vi "Lab3_ASK.vi"() -> ()   [LabVIEW 2019]
uses:
  <vilib>/addons/Modulation/Digital/General/MT Generate Bits (Galois, PN Order).vi
  <vilib>/addons/Modulation/Digital/Support/Common/Validators/mod_Generate Bits Validate.vi
  <vilib>/addons/Modulation/Analog/support/mod_Set Error Source.vi
  <vilib>/addons/Modulation/Digital/Support/Common/Validators/mod_AWGN Validate.vi
  <vilib>/addons/Modulation/Digital/Impairments/subVIs/mod_createSeeds.vi
  <vilib>/addons/Modulation/Digital/Support/Common/Validators/mod_Validate Samples Per Symbol.vi
  <vilib>/addons/Modulation/Analog/support/Validators/mod_Validate Complex Waveform.vi
  <vilib>/addons/Modulation/Analog/support/Validators/mod_WFErrorHandler.vi
  <vilib>/addons/Modulation/Digital/General/MT Generate ASK system parameters (M).vi
  <vilib>/addons/Modulation/Digital/General/subVIs/mod_Generate Bits PN Sequence.vi
  <vilib>/addons/Modulation/Digital/Support/Common/Validators/mod_Generate Filter Coefficients Validate.vi
  <vilib>/addons/Modulation/Digital/General/subVIs/mod_Generate Filter Coefficients.vi
  <vilib>/Analysis/1siggen.llb/Gaussian White Noise (obs 90).vi
  <vilib>/addons/Modulation/Analog/MT Upconvert Baseband (Real).vi
  <vilib>/addons/Modulation/niDMT.lvlib
  <vilib>/addons/Modulation/niAMT.lvlib
panel:
  out "Upconverted Wave":waveform(dbl)(graph)
  in  "Reset":bool=TRUE
  out "Waveform Graph":cluster{"t0":dbl, "dt":dbl, "Y":dbl[]}(graph)
  in  "Symbol Rate(HZ)":dbl format="%#_2p"
  in  "Carrier Freq(HZ)":dbl format="%#_2p"
  in  "pulse shaping filter":T1(ring)
  in  "M-ASK":u16(ring) items=["2"=2, "4"=4, "8"=8, "16"=16]
  in  "Eb/No(dB)":dbl
  in  "stop":bool
  out "ASK Constellation":T2(graph)
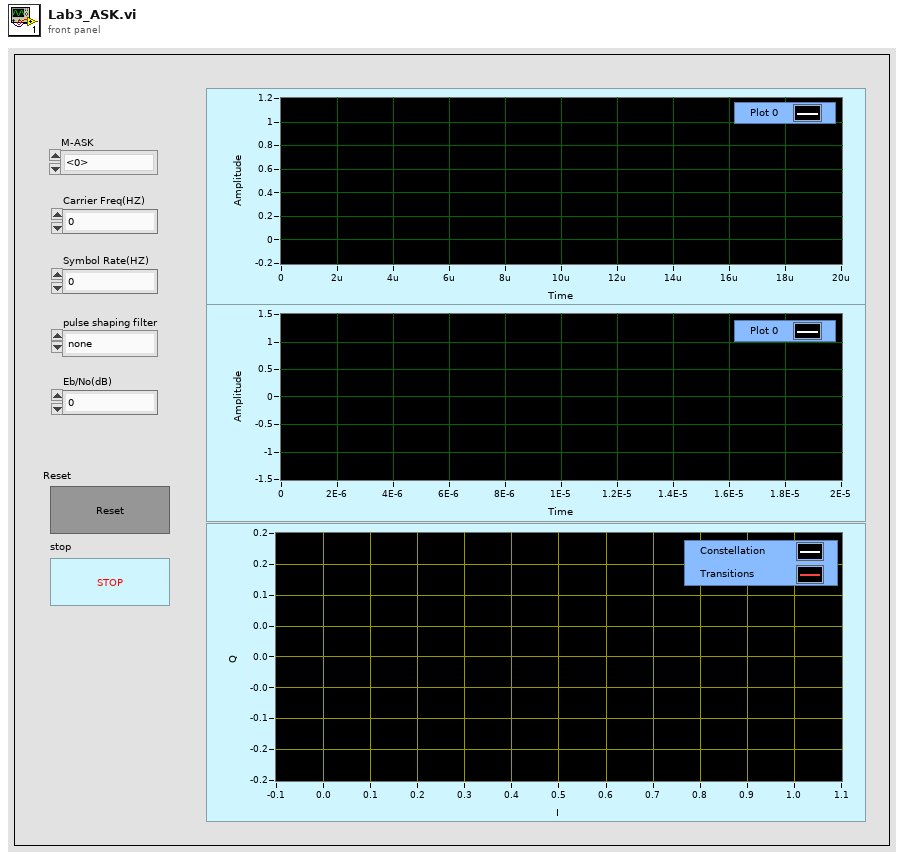
[diagram p1: front panel]
types:
  T1 = enum16{"none", "Raised Cosine", "Root Raised Cos", "Gaussian"}
  T2 = cluster{"Decimated Array":dbl[], "Decimated Array":dbl[]}[]
  T3 = enum16{"FSK", "PSK", "QAM", "MSK", "PAM", "ASK", "CPM"}
  T4 = cluster{"samples per symbol (16)":i32, "symbol map":cdb[]}
  T5 = typedef "niAMT.lvlib/Complex Data Waveform.ctl" = cluster{"t0":dbl, "dt":dbl, "Y":cdb[]}
  T6 = cluster{"constellation":dbl[], "oversampled data":dbl[]}[]
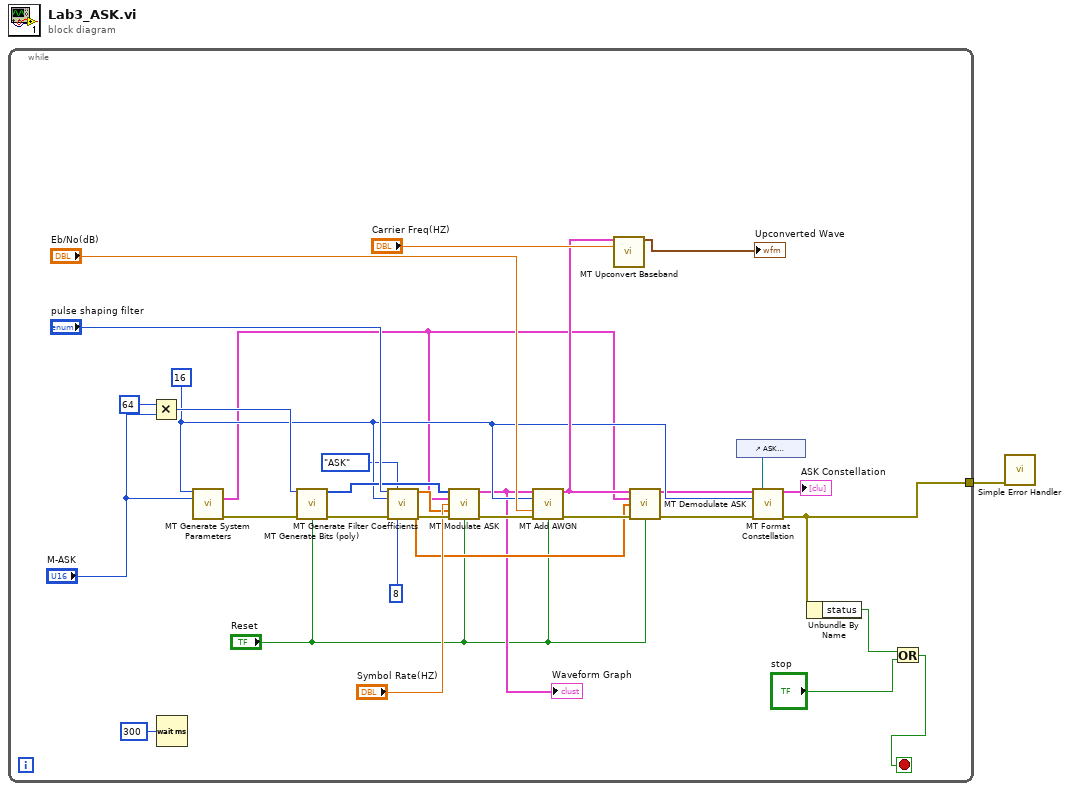
[diagram p0: block diagram]
diagram:
  n1 = while {
    tunnel: [w9] -> w1
    stop <- w6 stop-if-true
    w13 = 16 ("samples per symbol (16)")
    n2 = Multiply(x=u16 64, y="M-ASK") -> (x*y=w25:u16)
    n3 = Wait (ms)(milliseconds to wait=u32 300) -> ()  [unwired: 1 out]
    n4 = call-poly <vilib>:"MT Generate System Parameters.vi"("samples per symbol (16)"=w13, "M-ASK (2)"="M-ASK") -> ("ASK system parameters"=w12:T4, "error out"=w29:errorcluster)  [unwired: 11 in, 1 out]
    n5 = call-poly <vilib>:"MT Generate Bits (poly).vi"("total bits (128)"=w25, "error in (no error)"=w29, "reset? (T)"="Reset") -> ("output bit stream"=w14:i8[], "error out"=w28:errorcluster)  [unwired: 10 in, 1 out]
    n6 = call <vilib>:"MT Generate Filter Coefficients.vi"("pulse shaping filter (none)"="pulse shaping filter", "modulation type"=T3."ASK", "pulse shaping samples per symbol (16)"=w13, "error in (no error)"=w28, "filter length (symbols)"=8) -> ("pulse shaping filter coefficients"=w16:dbl[], "matched filter coefficients"=w17:dbl[], "error out"=w22:errorcluster)  [unwired: 8 in]
    n7 = call <vilib>:"MT Modulate ASK.vi"("input bit stream"=w14, "ASK system parameters"=w12, "symbol rate (Hz)"="Symbol Rate(HZ)", "pulse shaping filter coefficients"=w16, "error in (no error)"=w22, "reset? (T)"="Reset") -> ("output complex waveform"=w10:T5, "error out"=w21:errorcluster)  [unwired: 7 in, 1 out]
    "Waveform Graph" <- w10
    n8 = call <vilib>:"MT Add AWGN.vi"("input complex waveform"=w10, "samples per symbol (16)"=w13, "Eb/N0 (10 dB)"="Eb/No(dB)", "error in (no error)"=w21, "reset? (T)"="Reset") -> ("output complex waveform"=w19:T5, "error out"=w18:errorcluster)  [unwired: 8 in, 1 out]
    n9 = call-poly <vilib>:"MT Upconvert Baseband.vi"("baseband waveform (complex)"=w19, "carrier frequency (Hz)"="Carrier Freq(HZ)") -> ("passband waveform"=→"Upconverted Wave":waveform(dbl))  [unwired: 12 in, 1 out]
    n10 = call <vilib>:"MT Demodulate ASK.vi"("input complex waveform"=w19, "ASK system parameters"=w12, "matched filter coefficients"=w17, "error in (no error)"=w18, "reset? (T)"="Reset") -> ("recovered complex waveform"=w4:T5, "error out"=w3:errorcluster)  [unwired: 6 in, 3 out]
    n11 = control-ref of="ASK Constellation"() -> (w32:refnum<vi>)
    n12 = call <vilib>:"MT Format Constellation.vi"("waveform"=w4, "constellation reference"=w32, "samples per symbol"=w13, "error in (no error)"=w3) -> ("constellation graph"=→"ASK Constellation":T6, "error out"=w9:errorcluster)  [unwired: 1 in, 9 out]
    n13 = Unbundle By Name(w9) -> ("status"=w8:bool)
    n14 = Or(x=w8, y="stop") -> (x .or. y?=w6:bool)
  }
  n15 = call <vilib>:"Simple Error Handler.vi"("error in (no error)"=w1) -> ()  [unwired: 4 in, 5 out]
